vi "Modtag_Billede.vi"() -> ()   [LabVIEW 2018]
uses:
  <vilib>/myRIO/Instrument Drivers/Onboard IO/UART/typedef/VISA Configuration.ctl
  <vilib>/Instr/_visa.llb/VISA Configure Serial Port (Instr).vi
  <vilib>/myRIO/Express VI/Onboard IO/UART/UART Express VI.xnode
  <vilib>/myRIO/Instrument Drivers/Onboard IO/UART/UART.lvlib
panel:
  out "Intensity Graph 4":u8[][](graph)
  in  "Rotation \nOrientation":bool
  out "array":u8[](array[numeric])
  out "Picture recieved":u8[][](graph)
  out "Pixel array":u8[][](array[numeric])
  in  "stop":bool
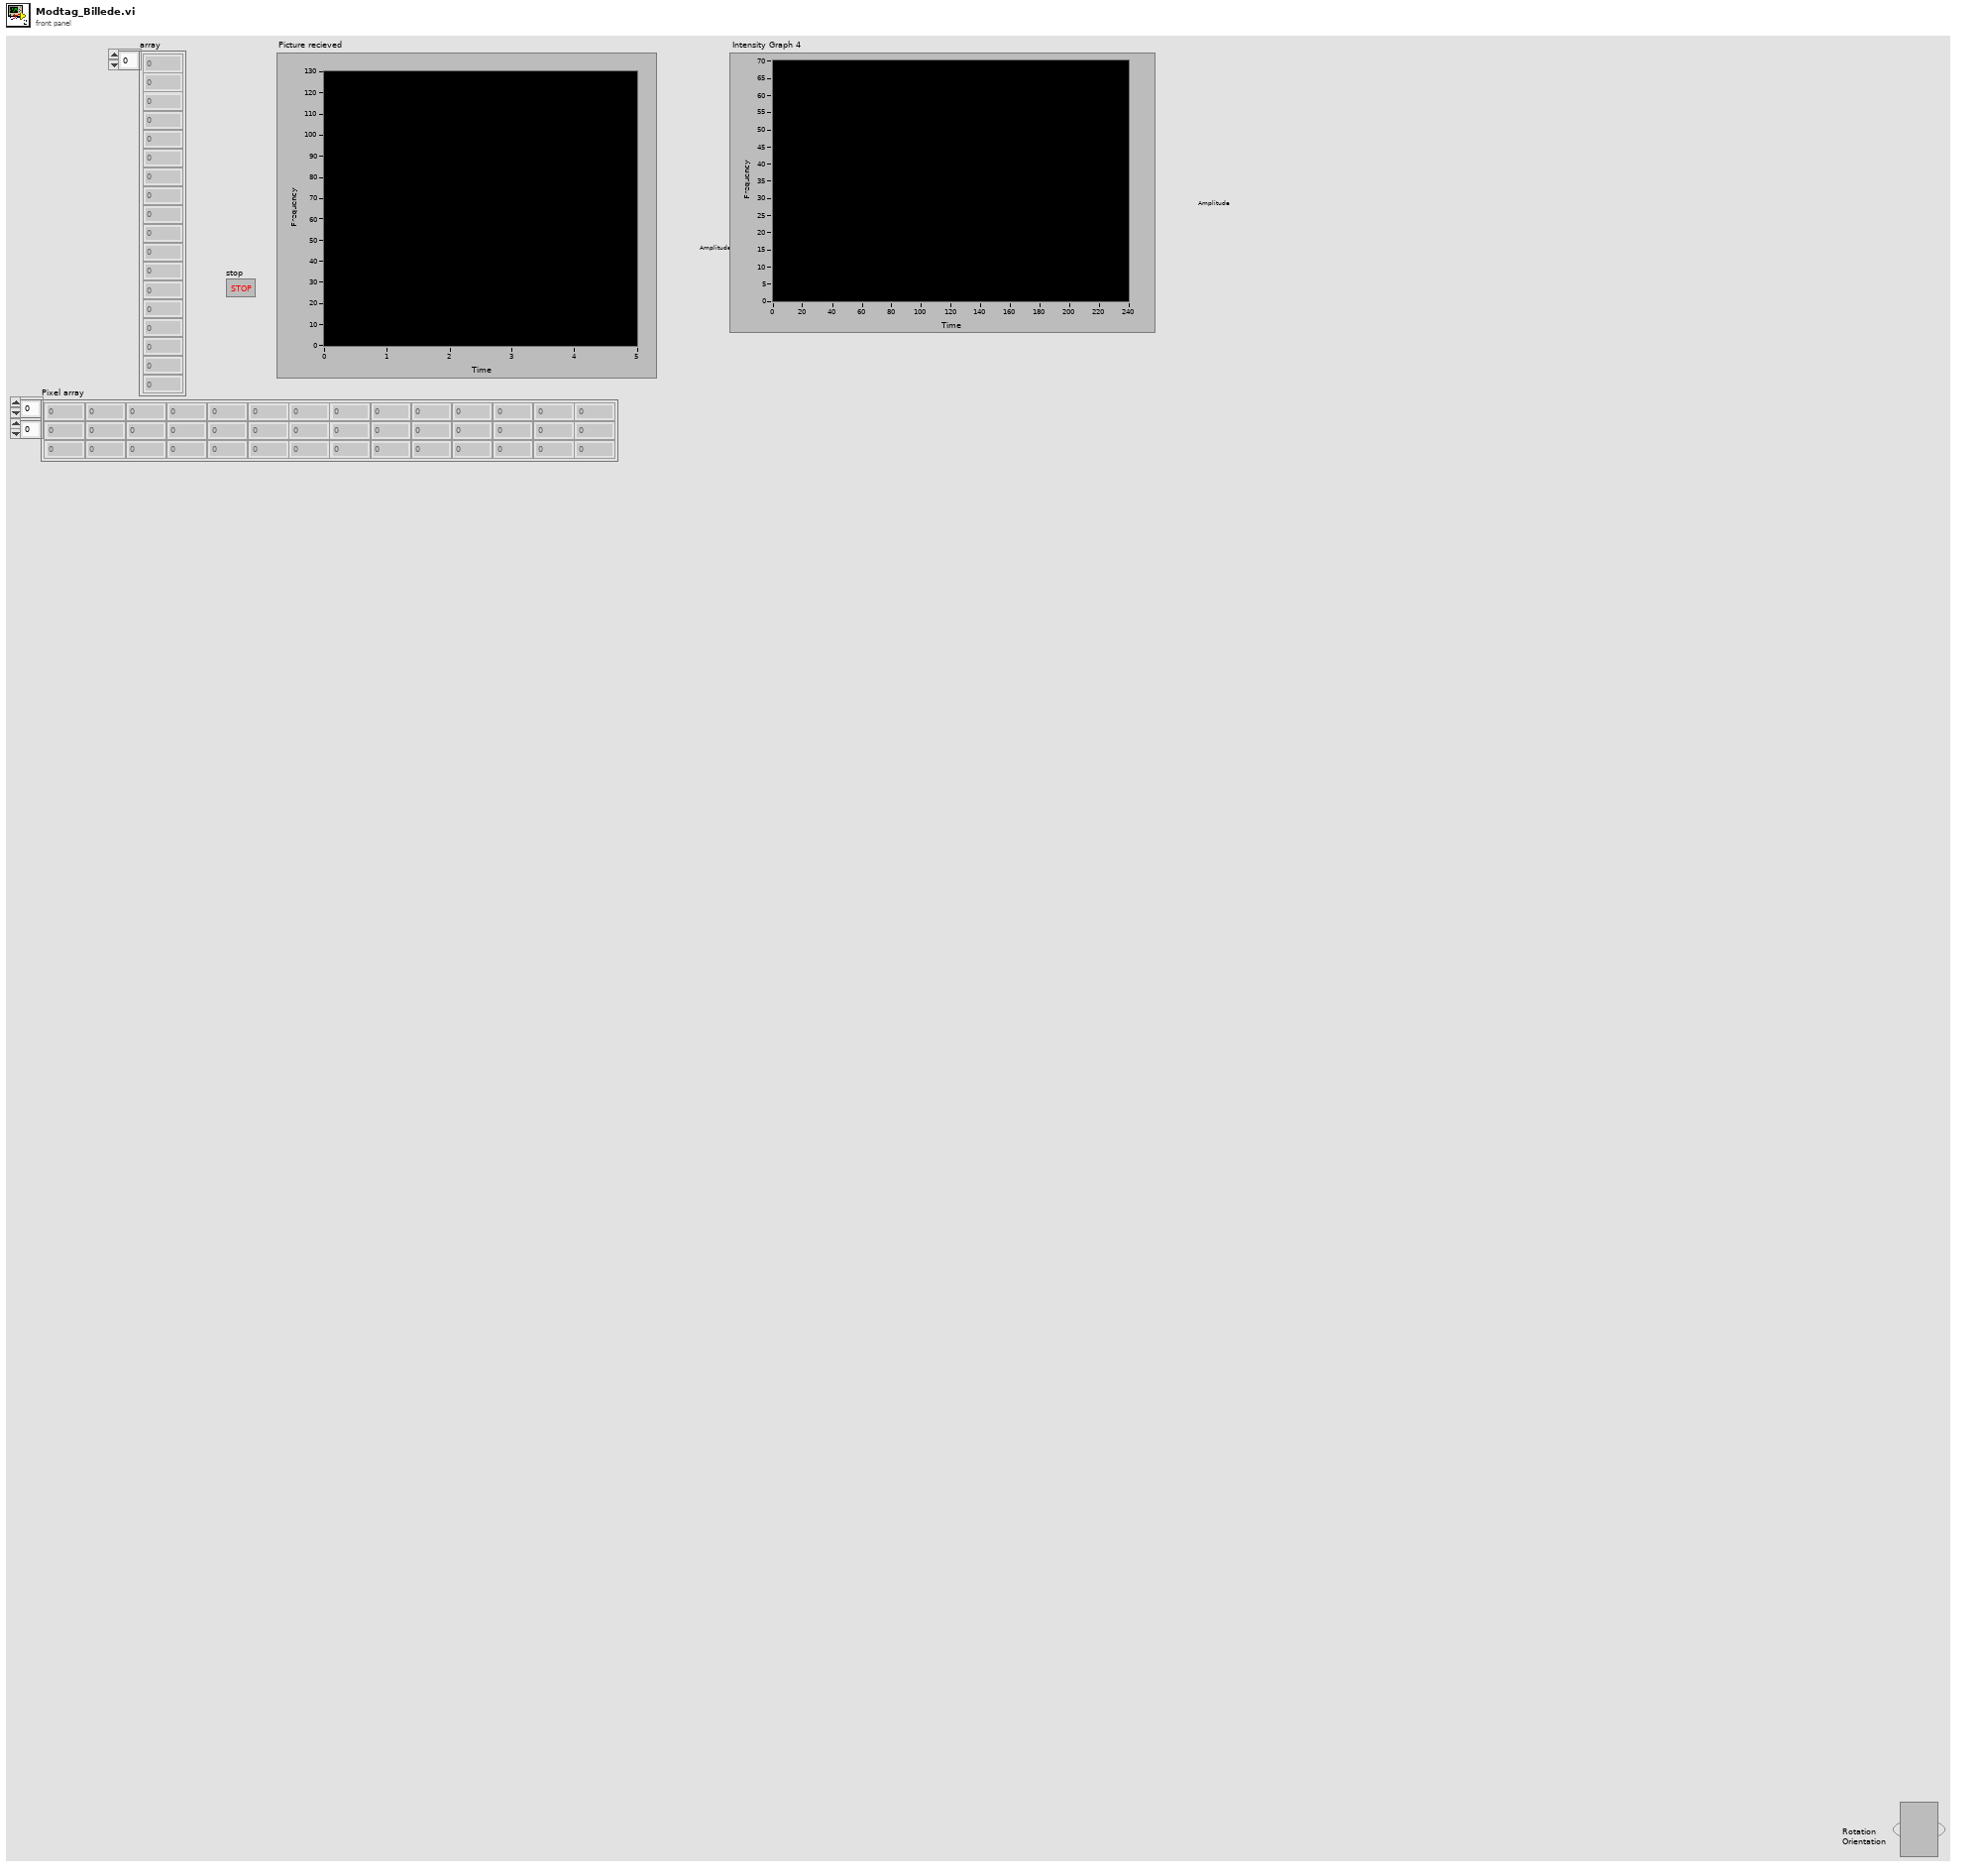
[diagram p1: front panel]
types:
  T1 = typedef "UART.lvlib/VISA Configuration.ctl" = cluster{"baud rate (9600)":u32, "data bits (8)":u16, "parity (0:none)":enum16{"None", "Odd", "Even", "Mark", "Space"}, "stop bits (10: 1 bit)":u16, "flow control (0:none)":u16, "termination char\n(0xA = '\\n' = LF) ":u8, "Enable Termination\nChar (T)":bool, "timeout (10sec)":u32}
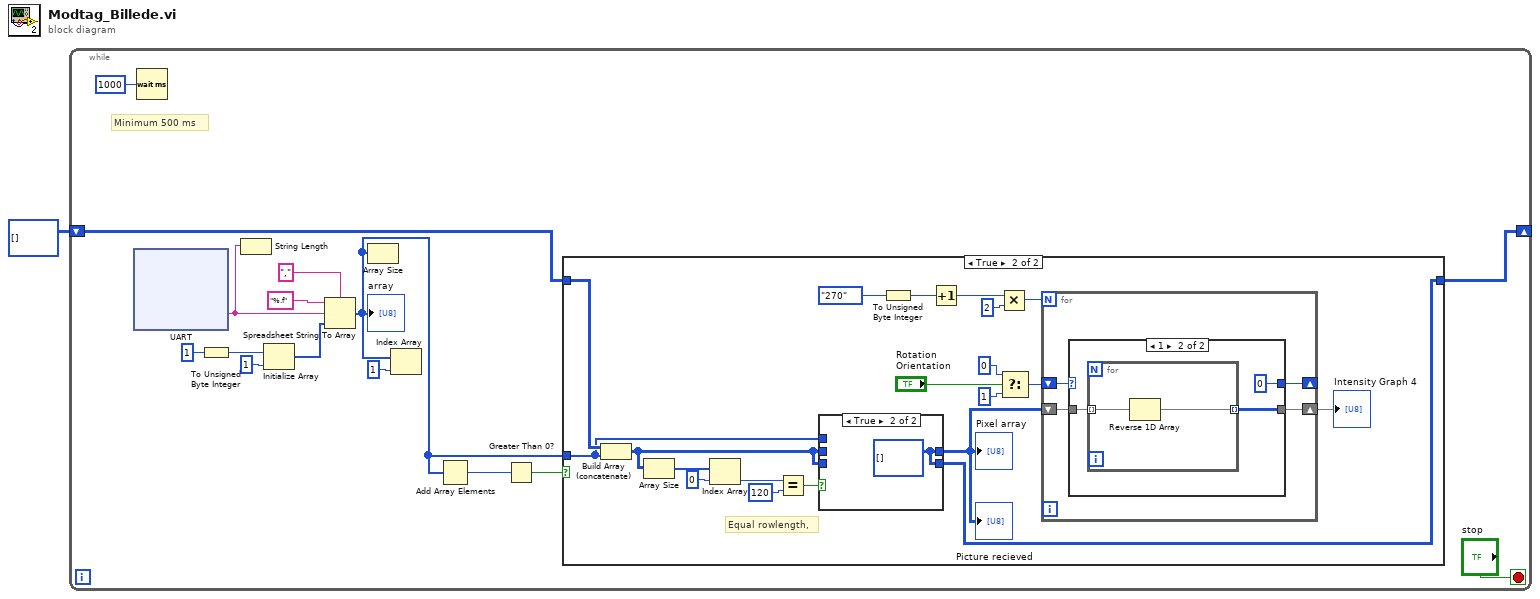
[diagram p0: block diagram]
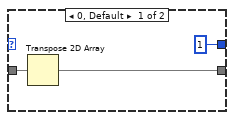
[diagram p3: hidden frame]
diagram:
  n1 = while {
    shift-right: [w10] -> _
    shift-left: u8[][] [] -> [w11]
    stop <- "stop" stop-if-true
    # "Minimum 500 ms"
    n2 = xnode "UART"() -> ("Characters Read"=w2:string)  [unwired: 1 in, 1 out]
    n3 = Wait (ms)(milliseconds to wait=u32 1000) -> ()  [unwired: 1 out]
    n4 = To Unsigned Byte Integer(number=u8 1) -> (unsigned 8bit integer=w8:u8)
    n5 = String Length(string=w2) -> ()  [unwired: 1 out]
    n6 = Initialize Array(w8, 1 ("dimension size")) -> (w5:u8[])
    n7 = Spreadsheet String To Array(delimiter (Tab)=",", format string="%.f", spreadsheet string=w2, array type (2D Dbl)=w5) -> (array=w3:u8[])
    "array" <- w3
    n8 = Array Size(array=w3) -> ()  [unwired: 1 out]
    n9 = Index Array(array=w3, index=1) -> ()  [unwired: 1 out]
    n10 = Add Array Elements(numeric array=w3) -> (sum=w13:u8)
    n11 = Greater Than 0?(x=w13) -> (x > 0?=w12:bool)
    n12 = case shown="True" w12 {
      tunnel: w3 -> [_ w31]
      tunnel: w11 -> [w17 w37]
      tunnel: [w17 w29] -> w10
      frame False {
      }
      frame True {
        # "Equal rowlength,"
        n13 = Build Array (concatenate)(w37, w31) -> (w30:u8[][])
        n14 = Array Size(array=w30) -> (size(s)=w36:i32[])
        n15 = Index Array(array=w36, index=0) -> (element=w34:i32)
        n16 = Equal?(x=w34, y=120) -> (x = y?=w32:bool)
        n17 = case shown="True" w32 {
          tunnel: w31 -> [_ _]
          tunnel: w30 -> [w51 _]
          tunnel: [w51 w52] -> w18
          tunnel: w30 -> [w50 _]
          tunnel: [w50 w52] -> w29
          frame False {
          }
          frame True {
            w52 = u8[][] []
          }
        }
        "Pixel array" <- w18
        "Picture recieved" <- w18
        n18 = To Unsigned Byte Integer(number=enum8{"90", "180", "270"}."270" ("Rotation")) -> (unsigned 8bit integer=w20:u8)
        n19 = Increment(x=w20) -> (x+1=w22:u8)
        n20 = Multiply(x=w22, y=u8 2) -> (x*y=w23:u8)
        n21 = Select(t=u8 0, s="Rotation \nOrientation", f=u8 1) -> (s? t:f=w24:u8)
        n22 = for {
          N: w23 -> [_]
          shift-right: [w40] -> w19
          shift-left: w18 -> [w41]
          shift-right: [w38] -> _
          shift-left: w24 -> [w39]
          n23 = case shown="1" w39 {
            tunnel: w41 -> [w43 w47]
            tunnel: [w44 w46] -> w40
            tunnel: [u8 1 u8 0] -> w38
            frame 0, Default {
              n24 = Transpose 2D Array(2D array=w43) -> (transposed array=w44:u8[][])
            }
            frame 1 {
              n25 = for {
                tunnel: w47 -> [w49] mode=indexing
                tunnel: [w48] -> w46 mode=indexing
                n26 = Reverse 1D Array(array=w49) -> (reversed array=w48:u8[])
              }
            }
          }
        }
        "Intensity Graph 4" <- w19
      }
    }
  }
